vi "Ask Wash Parameters.vi"(8 "error in (no error)":errorcluster, 10 "Car Option":string[](array[string]), 11 "Controller in":refnum<class "Controller.lvclass">) -> (0 "error out":errorcluster, 3 "Controller out":refnum<class "Controller.lvclass">)   [LabVIEW 2015, in "Controller.lvlib" / "Controller.lvclass"]
uses:
  Controller.lvclass
  Controller.lvclass/Controller.ctl
  Database/Database Messages/Read Config File Msg/Read Config File Msg.lvclass/Read Config File Msg.ctl
  <vilib>/ActorFramework/Message Enqueuer/Message Enqueuer.lvclass/Message Enqueuer.ctl
  <vilib>/ActorFramework/Message Enqueuer/Enqueue.vi
  <vilib>/ActorFramework/Message Priority Queue/Priority Enqueue.vi
  Database/Database Messages/Read Config File Msg/Read Config File Msg.lvclass
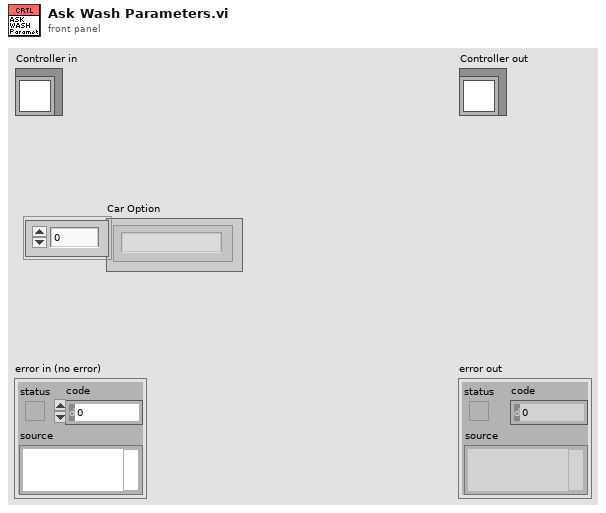
[diagram p1: front panel]
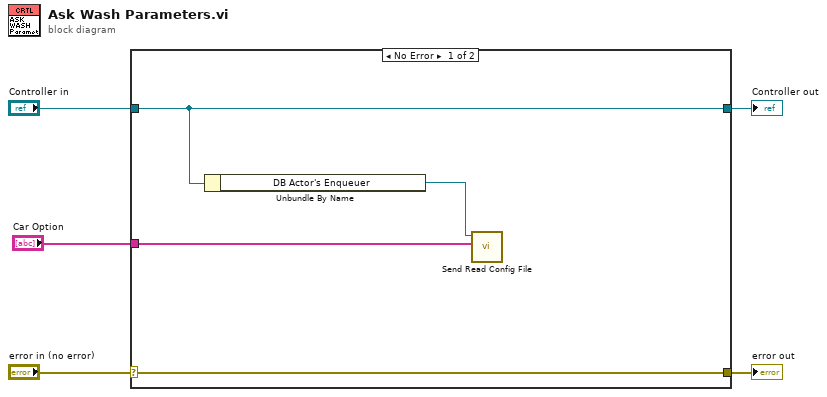
[diagram p0: block diagram]
diagram:
  n1 = case shown="No Error" "error in (no error)" {
    selector: "error in (no error)" -> [w9 w11]
    tunnel: [w9 w11] -> w4
    tunnel: [w8 w10] -> w2
    tunnel: "Controller in" -> [w8 w10]
    tunnel: "Car Option" -> [w6 _]
    frame No Error {
      n2 = Unbundle By Name(w8) -> ("DB Actor's Enqueuer"=w7:refnum<class "Message Enqueuer.lvclass">)
      n3 = call "Send Read Config File.vi"("Car Option"=w6, "Message Enqueuer"=w7) -> ()  [unwired: 8 in, 2 out]
    }
    frame Error {
    }
  }
  "error out" <- w4
  "Controller out" <- w2
